vi "布尔状态识别.vi"(9 "布尔名称":string, 10 "表格":string[][](array[string]), 11 "布尔":bool) -> (3 "布尔结果":bool)   [LabVIEW 2021]
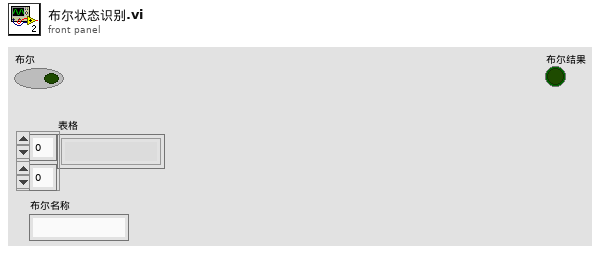
[diagram p1: front panel]
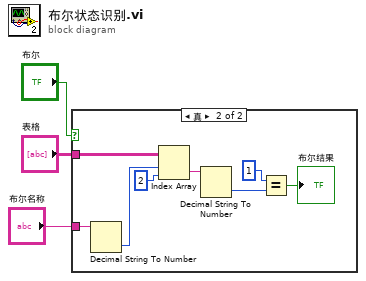
[diagram p0: block diagram]
diagram:
  n1 = case shown="真" "布尔" {
    tunnel: "表格" -> [_ w9]
    tunnel: "布尔名称" -> [_ w8]
    frame False {
    }
    frame True {
      n2 = Decimal String To Number(string=w8) -> (number=w10:i32)  [unwired: 2 in, 1 out]
      n3 = Index Array(array=w9, index (row)=w10, index (col)=2 ("禁用的索引 (列)")) -> (element=w7:string)
      n4 = Decimal String To Number(string=w7) -> (number=w6:i32)  [unwired: 2 in, 1 out]
      n5 = Equal?(x=1, y=w6) -> (x = y?=→"布尔结果":bool)
    }
  }
